vi "Sine_Trajectory_new2.vi"(4 "Frequency (Hz) 3":dbl, 6 "Frequency (Hz) 2":dbl, 7 "Amplitude":dbl, 8 "Offset":dbl, 9 "Frequency (Hz)":dbl, 10 "Duration (s)":dbl, 11 "Period (s)":dbl) -> (3 "Profile":cluster{"time (s)":dbl, "setpoint":dbl}[](array[cluster]) {"setpoint" format="%.2f"; "time (s)" format="%.3f"})   [LabVIEW 2015]
uses:
  <vilib>/Analysis/NI_AALBase.lvlib
panel:
  out "XY Graph":cluster{dbl, dbl}[](graph)
  # "Here needs to be 0.001 or so"
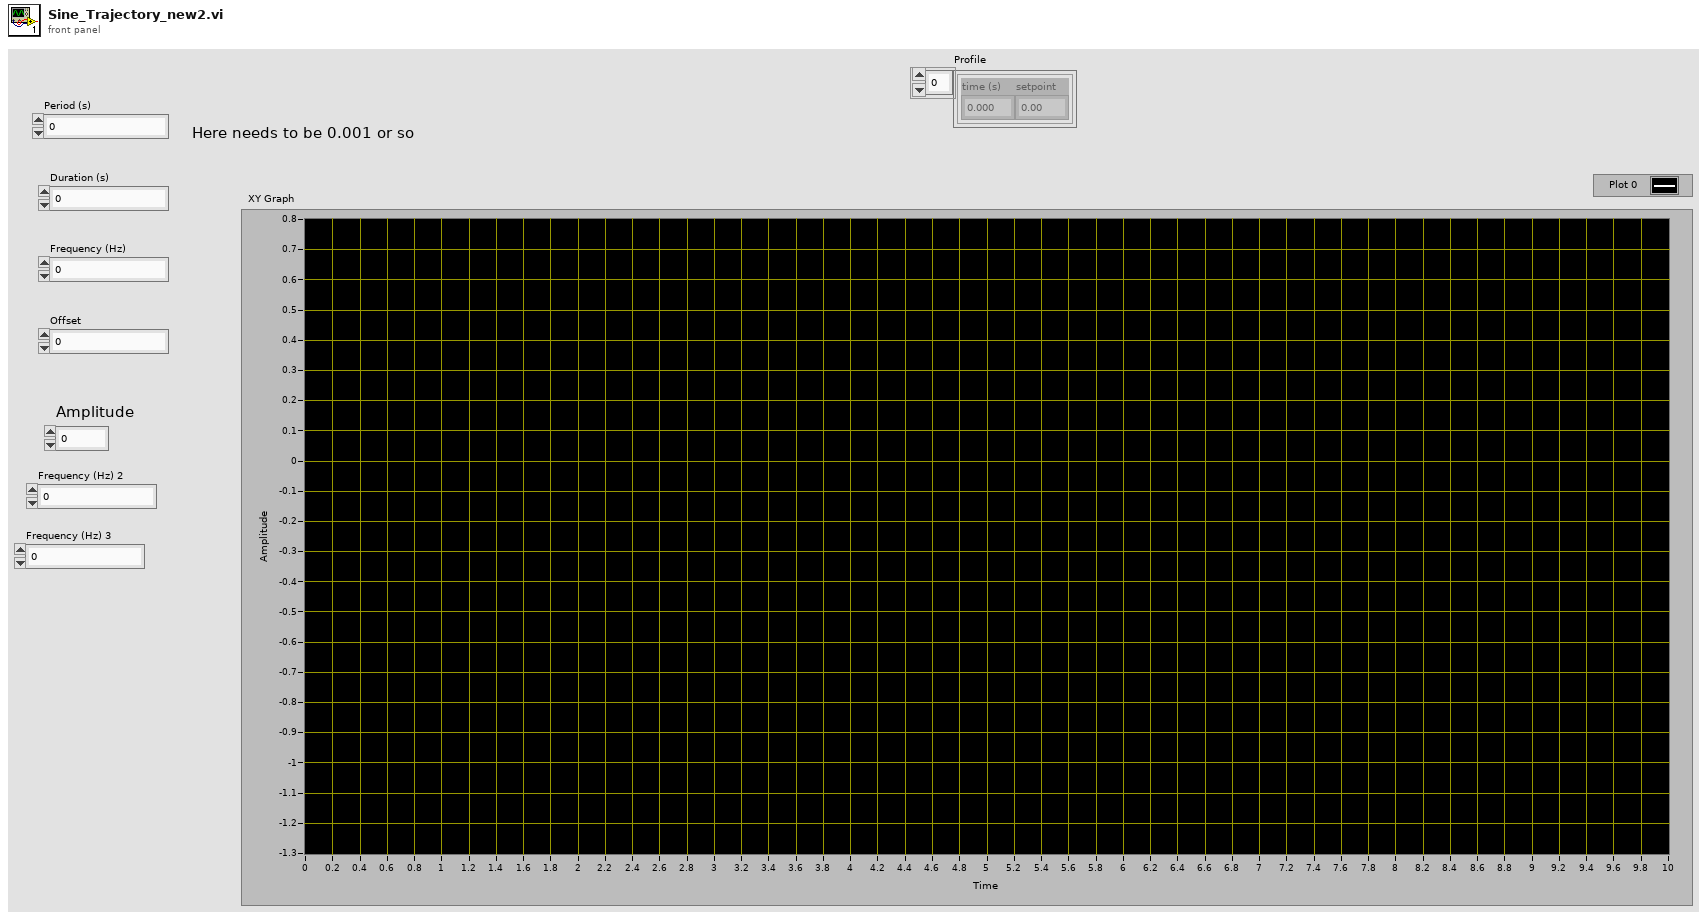
[diagram p1: front panel]
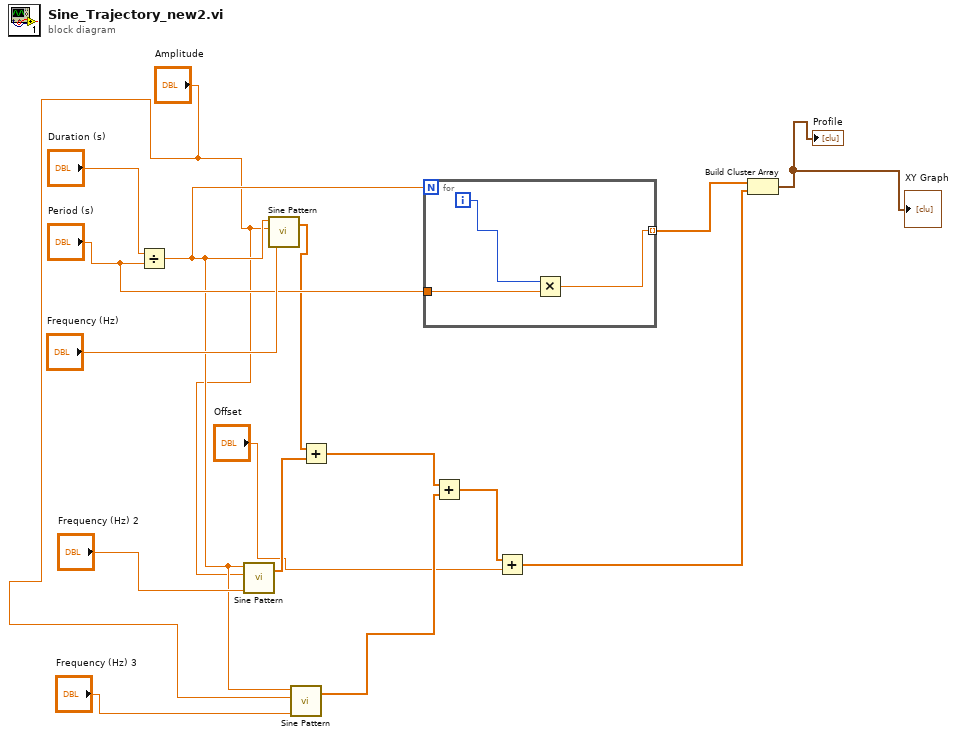
[diagram p0: block diagram]
diagram:
  n1 = Divide(x="Duration (s)", y="Period (s)") -> (x/y=w7:dbl)
  n2 = call <vilib>:"Sine Pattern.vi"("cycles"="Frequency (Hz) 2", "amplitude"="Amplitude", "samples"=w7) -> ("Sinusoidal Pattern"=w3:dbl[])  [unwired: 1 in, 1 out]
  n3 = call <vilib>:"Sine Pattern.vi"("cycles"="Frequency (Hz)", "amplitude"="Amplitude", "samples"=w7) -> ("Sinusoidal Pattern"=w11:dbl[])  [unwired: 1 in, 1 out]
  n4 = call <vilib>:"Sine Pattern.vi"("cycles"="Frequency (Hz) 3", "amplitude"="Amplitude", "samples"=w7) -> ("Sinusoidal Pattern"=w2:dbl[])  [unwired: 1 in, 1 out]
  n5 = Add(x=w11, y=w3) -> (x+y=w9:dbl[])
  n6 = for {
    N: w7 -> [_]
    tunnel: [w17] -> w14 mode=indexing
    tunnel: "Period (s)" -> [w19]
    i -> [w18]
    n7 = Multiply(x=w18, y=w19) -> (x*y=w17:dbl)
  }
  n8 = Add(x=w9, y=w2) -> (x+y=w5:dbl[])
  n9 = Add(x=w5, y="Offset") -> (x+y=w4:dbl[])
  n10 = Build Cluster Array(w14, w4) -> (→"XY Graph" →"Profile":cluster{dbl, dbl}[])
